vi "Modulation.vi"(0 "appended path":path, 1 "scramble_data":dbl[](array[numeric]), 2 "prb_num":dbl, 3 "module_type":dbl, 4 "error in (no error)":errorcluster caption="错误输入（无错误）") -> (5 "mod_data":cdb[](array[numeric]), 6 "error out":errorcluster caption="错误输出")   [LabVIEW 2015]
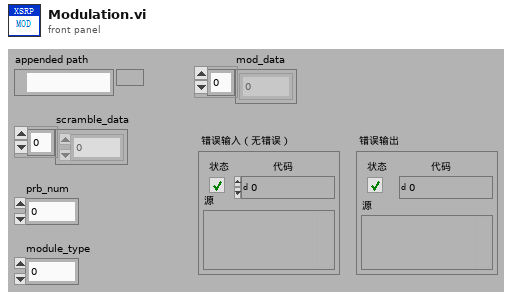
[diagram p1: front panel]
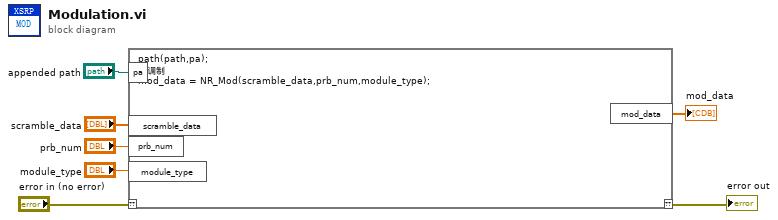
[diagram p0: block diagram]
diagram:
  n1 = script code="path(path,pa);\n%调制\nmod_data = NR_Mod(scramble_data,prb_num,module_type);"("??"="error in (no error)", "pa"="appended path", "scramble_data"="scramble_data", "prb_num"="prb_num", "module_type"="module_type") -> ("??"=→"error out":errorcluster, "mod_data"=→"mod_data":cdb[])
